vi "Solution part 1a.vi"(11 "data?":bool) -> (3 "Occupied seats (result)":i16)   [LabVIEW 2020]
uses:
  Direction.ctl
panel:
  out "Rounds":i32
  out "Seats":string[](array[string])
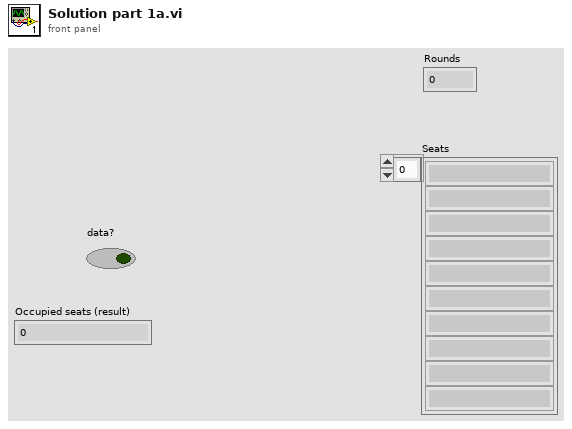
[diagram p1: front panel]
types:
  T1 = typedef "Direction.ctl" = cluster{"x":i32, "y":i32}
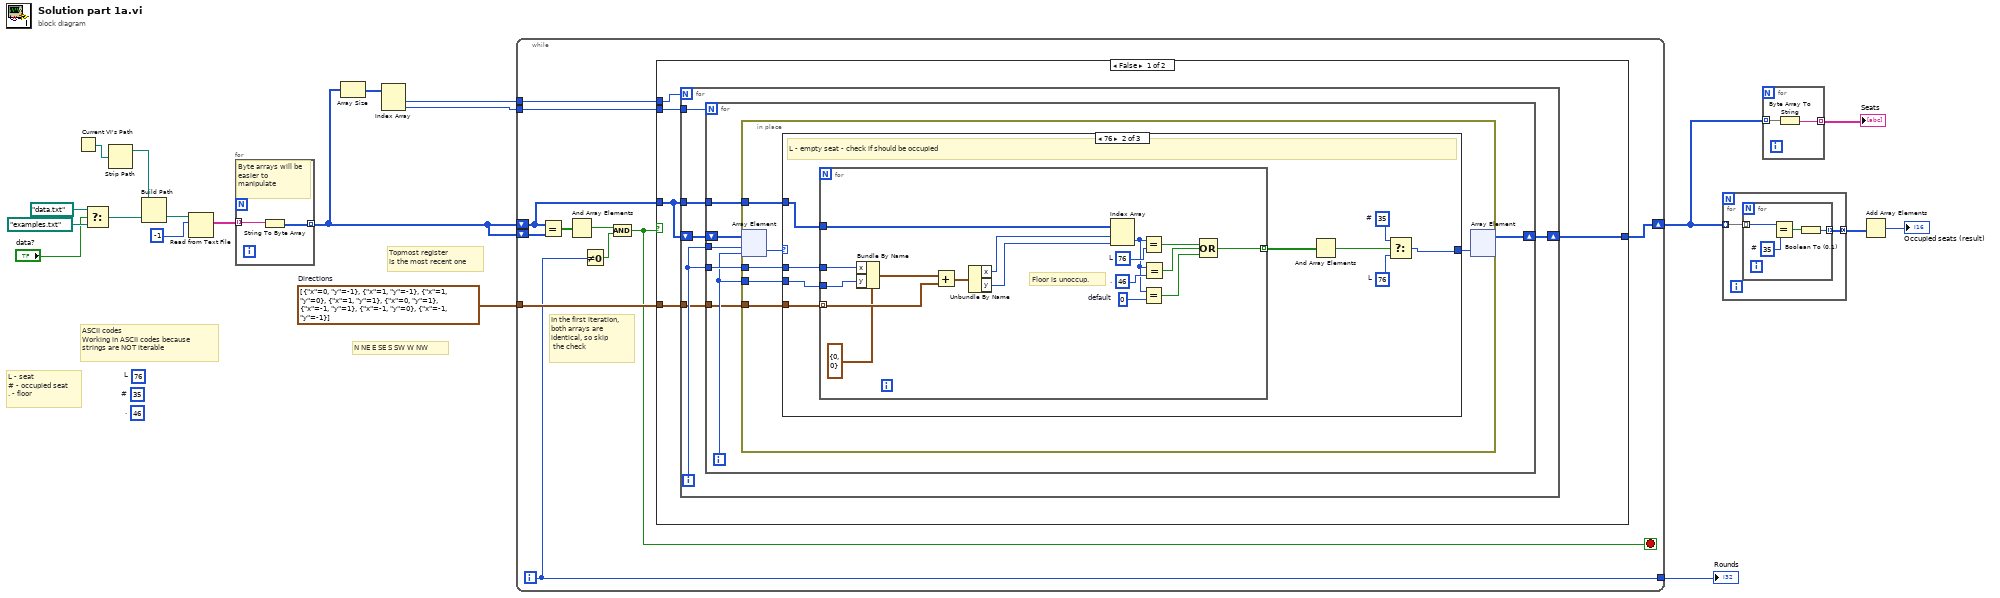
[diagram p0: block diagram]
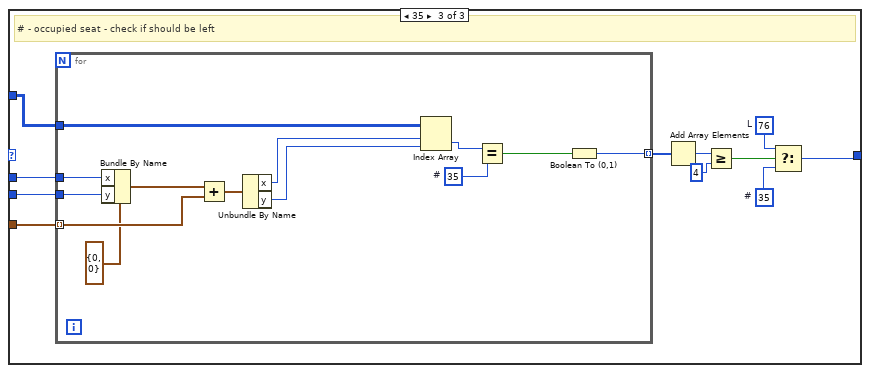
[diagram p3: hidden frame]
diagram:
  w1 = T1[] [{"x"=0, "y"=-1}, {"x"=1, "y"=-1}, {"x"=1, "y"=0}, {"x"=1, "y"=1}, {"x"=0, "y"=1}, {"x"=-1, "y"=1}, {"x"=-1, "y"=0}, {"x"=-1, "y"=-1}]  # Directions
  (unwired) u8 76  # L
  (unwired) u8 46  # .
  (unwired) u8 35  # #
  # "N NE E SE S SW W NW"
  # "ASCII codes\nWorking in ASCII codes because\nstrings are NOT iterable"
  # "Topmost register\nis the most recent one"
  # "L - seat\n# - occupied seat\n. - floor"
  n1 = Current VI's Path() -> (path=w16:path)
  n2 = Select(t=path "data.txt", s="data?", f=path "examples.txt") -> (s? t:f=w17:path)
  n3 = Strip Path(path=w16) -> (stripped path=w15:path)  [unwired: 1 out]
  n4 = Build Path(base path=w15, name or relative path=w17) -> (appended path=w14:path)
  n5 = Read from Text File(file (use dialog)=w14, count=-1) -> (text=w11:string[])  [unwired: 2 in, 3 out]
  n6 = for {
    tunnel: w11 -> [w21] mode=indexing
    tunnel: [w20] -> w3 mode=indexing
    # "Byte arrays will be easier to manipulate"
    n7 = String To Byte Array(string=w21) -> (unsigned byte array=w20:u8[])
  }
  n8 = Array Size(array=w3) -> (size(s)=w10:i32[])
  n9 = Index Array(array=w10) -> (element #1=w6:i32, element #2=w7:i32)  [unwired: 2 in]
  n10 = while {
    shift-right: [w30] -> w5
    shift-left: w3 -> [w31]
    shift-left: w3 -> [w22]
    tunnel: w6 -> [w29]
    tunnel: w7 -> [w28]
    tunnel: w1 -> [w27]
    tunnel: [w23] -> w2
    i -> [w23]
    stop <- w25 stop-if-true
    # "In the first iteration,\nboth arrays are \nidentical, so skip\n the check"
    n11 = Equal?(x=w22, y=w31) -> (x = y?=w32:bool[][])
    n12 = And Array Elements(Boolean array=w32) -> (logical AND=w26:bool)
    n13 = Not Equal To 0?(x=w23) -> (x != 0?=w24:bool)
    n14 = And(x=w26, y=w24) -> (x .and. y?=w25:bool)
    n15 = case shown="False" w25 {
      tunnel: w22 -> [w33 w108]
      tunnel: [w37 w108] -> w30
      tunnel: w29 -> [w35 _]
      tunnel: w28 -> [w34 _]
      tunnel: w27 -> [w36 _]
      frame False {
        n16 = for {
          N: w35 -> [_]
          tunnel: w34 -> [w42]
          shift-right: [w41] -> w37
          shift-left: w33 -> [w43]
          tunnel: w36 -> [w39]
          tunnel: w33 -> [w38]
          i -> [w40]
          n17 = for {
            N: w42 -> [_]
            tunnel: w40 -> [w50]
            shift-right: [w49] -> w41
            shift-left: w43 -> [w48]
            tunnel: w40 -> [w47]
            tunnel: w39 -> [w45]
            tunnel: w38 -> [w44]
            i -> [w46]
            n18 = in-place {
              in-place-border: w44 -> [w54]
              in-place-border: w47 -> [w53]
              in-place-border: w46 -> [w52]
              in-place-border: w45 -> [w51]
              n19 = in-place-array #1(w48, w50, w46) -> (w56:u8)
              n20 = case shown="76" w56 {
                selector: w56 -> [w57 _ _]
                tunnel: [w57 w59 w86] -> w55
                tunnel: w54 -> [_ w65 w93]
                tunnel: w53 -> [_ w64 w92]
                tunnel: w52 -> [_ w63 w91]
                tunnel: w51 -> [_ w66 w94]
                frame 46, Default {
                  # ". - Floor - skip"
                }
                frame 76 {
                  w60 = u8 35  # #
                  w61 = u8 76  # L
                  # "L - empty seat - check if should be occupied"
                  n21 = for {
                    tunnel: w66 -> [w83] mode=indexing
                    tunnel: w65 -> [w82]
                    tunnel: w64 -> [w79]
                    tunnel: w63 -> [w78]
                    tunnel: [w67] -> w58 mode=indexing
                    w69 = u8 0  # default
                    w75 = u8 46  # .
                    w77 = u8 76  # L
                    # "Floor is unoccup."
                    n22 = Bundle By Name(cluster=T1 {"x"=0, "y"=0} ("Direction"), "x"=w79, "y"=w78) -> (w81:T1)
                    n23 = Add(x=w81, y=w83) -> (x+y=w70:T1)
                    n24 = Unbundle By Name(w70) -> ("x"=w74:i32, "y"=w73:i32)
                    n25 = Index Array(array=w82, index (row)=w74, index (col)=w73) -> (element=w68:u8)
                    n26 = Equal?(x=w68, y=w77) -> (x = y?=w72:bool)
                    n27 = Equal?(x=w68, y=w69) -> (x = y?=w71:bool)
                    n28 = Equal?(x=w68, y=w75) -> (x = y?=w76:bool)
                    n29 = Compound Arithmetic op=OR(w72, w76, w71) -> (w67:bool)
                  }
                  n30 = And Array Elements(Boolean array=w58) -> (logical AND=w62:bool)
                  n31 = Select(t=w60, s=w62, f=w61) -> (s? t:f=w59:u8)
                }
                frame 35 {
                  w85 = u8 76  # L
                  w90 = u8 35  # #
                  # "# - occupied seat - check if should be left"
                  n32 = for {
                    tunnel: w94 -> [w107] mode=indexing
                    tunnel: w93 -> [w106]
                    tunnel: w92 -> [w103]
                    tunnel: w91 -> [w102]
                    tunnel: [w95] -> w84 mode=indexing
                    w97 = u8 35  # #
                    n33 = Bundle By Name(cluster=T1 {"x"=0, "y"=0} ("Direction"), "x"=w103, "y"=w102) -> (w105:T1)
                    n34 = Add(x=w105, y=w107) -> (x+y=w99:T1)
                    n35 = Unbundle By Name(w99) -> ("x"=w101:i32, "y"=w100:i32)
                    n36 = Index Array(array=w106, index (row)=w101, index (col)=w100) -> (element=w98:u8)
                    n37 = Equal?(x=w98, y=w97) -> (x = y?=w96:bool)
                    n38 = Boolean To (0,1)(Boolean=w96) -> (0, 1=w95:i16)
                  }
                  n39 = Add Array Elements(numeric array=w84) -> (sum=w89:i16)
                  n40 = Greater Or Equal?(x=w89, y=i16 4) -> (x >= y?=w87:bool)
                  n41 = Select(t=w85, s=w87, f=w90) -> (s? t:f=w86:u8)
                }
              }
              n42 = in-place-array #1(w55) -> (w49:u8[][])  [unwired: 2 out]
            }
          }
        }
      }
      frame True {
      }
    }
  }
  "Rounds" <- w2
  n43 = for {
    tunnel: w5 -> [w110] mode=indexing
    tunnel: [w109] -> w9 mode=concatenating
    n44 = for {
      tunnel: w110 -> [w114] mode=indexing
      tunnel: [w112] -> w109 mode=indexing
      w111 = u8 35  # #
      n45 = Equal?(x=w114, y=w111) -> (x = y?=w113:bool)
      n46 = Boolean To (0,1)(Boolean=w113) -> (0, 1=w112:i16)
    }
  }
  n47 = for {
    tunnel: w5 -> [w116] mode=indexing
    tunnel: [w115] -> w4 mode=indexing
    n48 = Byte Array To String(unsigned byte array=w116) -> (string=w115:string)
  }
  "Seats" <- w4
  n49 = Add Array Elements(numeric array=w9) -> (sum=→"Occupied seats (result)":i16)
